vi "ABB Size 1D array.vi"(5 "Type":enum16{"Integer", "DBL", "STRING", "BOOLEAN"}(ring), 6 "Default":T1 {"Dbl" format="%.2f"}, 7 "Size":i32, 8 "Boolean Array in":bool[](array[boolean]), 9 "String Array in":string[](array[string]), 10 "DBL Array In":dbl[](array[numeric]) format="%.2f", 11 "Integer Array In":i32[](array[numeric])) -> (0 "Boolean Array out":bool[](array[boolean]), 1 "String Array out":string[](array[string]), 2 "DBL Array out":dbl[](array[numeric]) format="%.2f", 3 "Integer Array Out":i32[](array[numeric]))   [LabVIEW 2017]
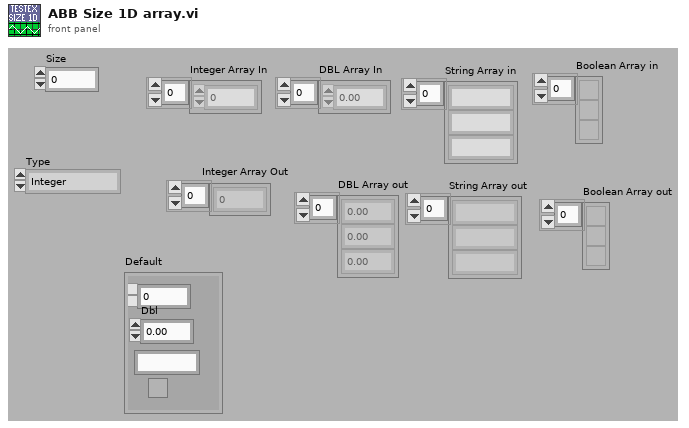
[diagram p1: front panel]
types:
  T1 = cluster{"Integer":i32, "Dbl":dbl, "String":string, "Boolean":bool}
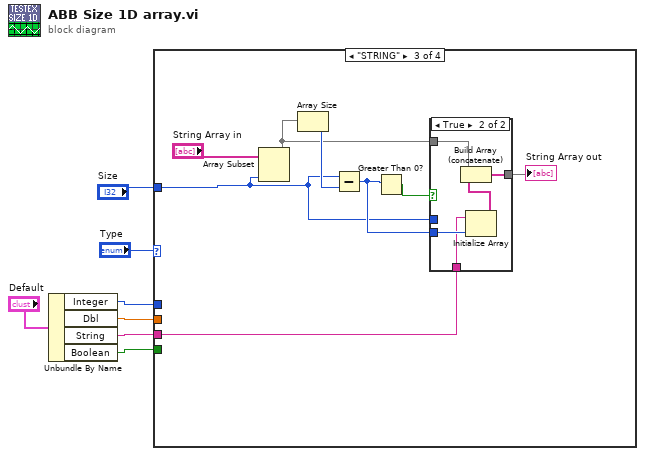
[diagram p0: block diagram]
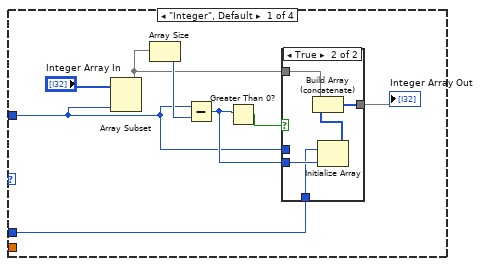
[diagram p2: hidden frame]
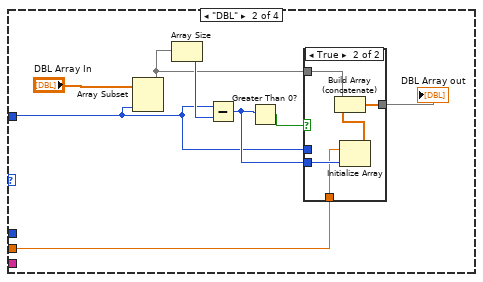
[diagram p4: hidden frame]
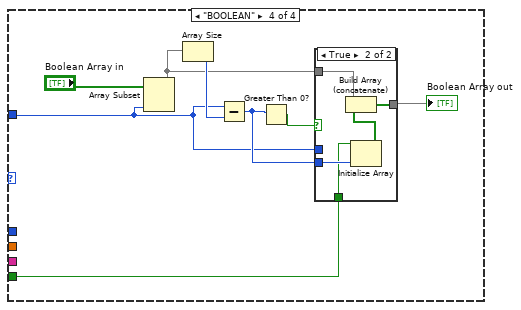
[diagram p7: hidden frame]
diagram:
  n1 = Unbundle By Name("Default") -> ("Integer"=w3:i32, "Dbl"=w4:dbl, "String"=w2:string, "Boolean"=w1:bool)
  n2 = case shown="\"STRING\"" "Type" {
    tunnel: "Size" -> [w11 w22 w36 w50]
    tunnel: w4 -> [_ w23 _ _]
    tunnel: w3 -> [w8 _ _ _]
    tunnel: w2 -> [_ _ w37 _]
    tunnel: w1 -> [_ _ _ w51]
    frame "Integer", Default {
      n3 = Array Subset(array="Integer Array In", length=w11) -> (w10:i32[])  [unwired: 1 in]
      n4 = Array Size(array=w10) -> (size(s)=w14:i32)
      n5 = Subtract(x=w11, y=w14) -> (x-y=w12:i32)
      n6 = Greater Than 0?(x=w12) -> (x > 0?=w13:bool)
      n7 = case shown="True" w13 {
        tunnel: w12 -> [_ w21]
        tunnel: w11 -> [_ _]
        tunnel: w10 -> [w16 w20]
        tunnel: [w16 w18] -> w9
        tunnel: w8 -> [_ w17]
        frame False {
        }
        frame True {
          n8 = Initialize Array(w17, w21) -> (w19:i32[])
          n9 = Build Array (concatenate)(w20, w19) -> (w18:i32[])
        }
      }
      "Integer Array Out" <- w9
    }
    frame "DBL" {
      n10 = Array Subset(array="DBL Array In", length=w22) -> (w26:dbl[])  [unwired: 1 in]
      n11 = Array Size(array=w26) -> (size(s)=w29:i32)
      n12 = Subtract(x=w22, y=w29) -> (x-y=w27:i32)
      n13 = Greater Than 0?(x=w27) -> (x > 0?=w28:bool)
      n14 = case shown="True" w28 {
        tunnel: w27 -> [_ w35]
        tunnel: w22 -> [_ _]
        tunnel: w26 -> [w30 w34]
        tunnel: [w30 w32] -> w24
        tunnel: w23 -> [_ w31]
        frame False {
        }
        frame True {
          n15 = Initialize Array(w31, w35) -> (w33:dbl[])
          n16 = Build Array (concatenate)(w34, w33) -> (w32:dbl[])
        }
      }
      "DBL Array out" <- w24
    }
    frame "STRING" {
      n17 = Array Subset(array="String Array in", length=w36) -> (w40:string[])  [unwired: 1 in]
      n18 = Array Size(array=w40) -> (size(s)=w43:i32)
      n19 = Subtract(x=w36, y=w43) -> (x-y=w41:i32)
      n20 = Greater Than 0?(x=w41) -> (x > 0?=w42:bool)
      n21 = case shown="True" w42 {
        tunnel: w41 -> [_ w49]
        tunnel: w36 -> [_ _]
        tunnel: w40 -> [w44 w48]
        tunnel: [w44 w46] -> w39
        tunnel: w37 -> [_ w45]
        frame False {
        }
        frame True {
          n22 = Initialize Array(w45, w49) -> (w47:string[])
          n23 = Build Array (concatenate)(w48, w47) -> (w46:string[])
        }
      }
      "String Array out" <- w39
    }
    frame "BOOLEAN" {
      n24 = Array Subset(array="Boolean Array in", length=w50) -> (w54:bool[])  [unwired: 1 in]
      n25 = Array Size(array=w54) -> (size(s)=w57:i32)
      n26 = Subtract(x=w50, y=w57) -> (x-y=w55:i32)
      n27 = Greater Than 0?(x=w55) -> (x > 0?=w56:bool)
      n28 = case shown="True" w56 {
        tunnel: w55 -> [_ w63]
        tunnel: w50 -> [_ _]
        tunnel: w54 -> [w58 w62]
        tunnel: [w58 w60] -> w52
        tunnel: w51 -> [_ w59]
        frame False {
        }
        frame True {
          n29 = Initialize Array(w59, w63) -> (w61:bool[])
          n30 = Build Array (concatenate)(w62, w61) -> (w60:bool[])
        }
      }
      "Boolean Array out" <- w52
    }
  }
